vi "ttlpuls.vi"(0 "lines":tag="Dev1/port2/line7", 1 "Pause Time (ms)":u32=2000, 2 "Pulse Length (ms)":u32=300, 3 "Number of Pulses":i32=5) -> ()   [LabVIEW 2011]
uses:
  <vilib>/DAQmx/write.llb/DAQmx Write (Digital 1D Bool 1Chan 1Samp).vi
  <vilib>/DAQmx/create/channels.llb/DAQmx Create Channel (DO-Digital Output).vi
  <vilib>/DAQmx/miscellaneous.llb/DAQmx Fill In Error Info.vi
  Program Files/National Instruments/LabVIEW 2011/resource/objmgr/daqmx.rc
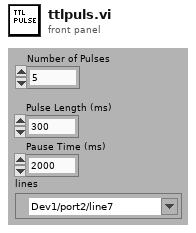
[diagram p1: front panel]
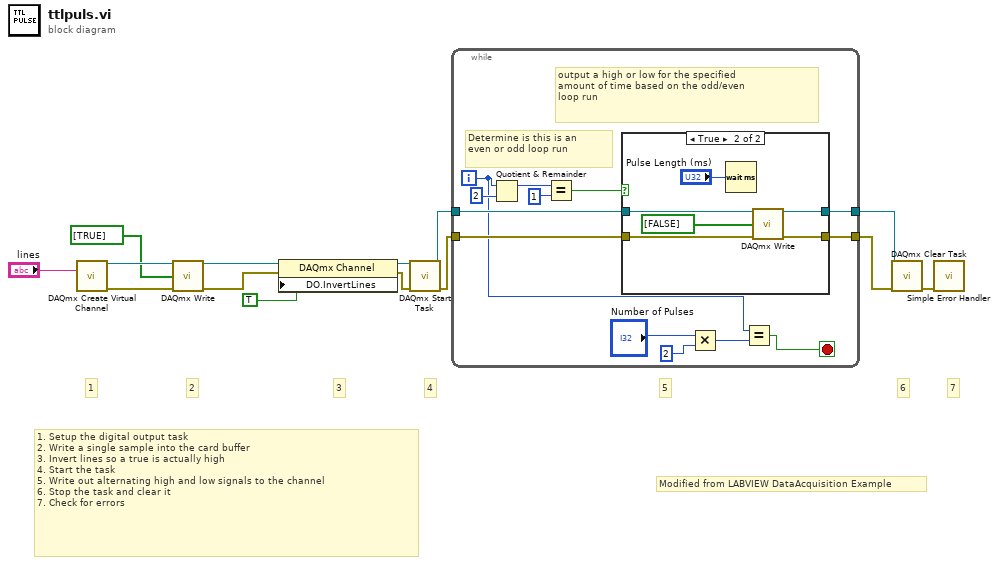
[diagram p0: block diagram]
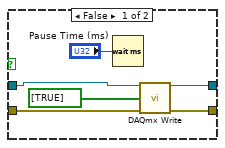
[diagram p2: hidden frame]
diagram:
  # "Modified from LABVIEW DataAcquisition Example"
  # "5"
  # "1. Setup the digital output task\n2. Write a single sample into the card buffer\n3. Invert lines so a true is actually high\n4. Start the task\n5. Write out alternating high and low signals to the channel\n6. Stop the task and clear it\n7. Check for errors"
  # "7"
  # "6"
  # "4"
  # "3"
  # "2"
  # "1"
  n1 = call-poly <vilib>:"DAQmx Create Virtual Channel.vi"("lines"="lines") -> ("task out"=w14:refnum<k21>, "error out"=w13:errorcluster)  [unwired: 13 in]
  n2 = call-poly <vilib>:"DAQmx Write.vi"("task/channels in"=w14, "data"=bool[] [TRUE], "error in"=w13) -> ("task out"=w5:refnum<k21>, "error out"=w1:errorcluster)  [unwired: 10 in, 1 out]
  n3 = property class="DAQmx Channel"(reference=w5, error in=w1, "DO.InvertLines"=TRUE) -> (reference out=w4:refnum<k21>, error out=w3:errorcluster)
  n4 = call <vilib>:"DAQmx Start Task.vi"("task/channels in"=w4, "error in"=w3) -> ("task out"=w12:refnum<k21>, "error out"=w11:errorcluster)  [unwired: 12 in]
  n5 = while {
    tunnel: w12 -> [w27]
    tunnel: w11 -> [w26]
    tunnel: [w25] -> w10
    tunnel: [w24] -> w9
    i -> [w18]
    stop <- w19 stop-if-true
    # "output a high or low for the specified\namount of time based on the odd/even\nloop run"
    # "Determine is this is an\neven or odd loop run"
    n6 = Quotient & Remainder(x=w18, y=2) -> (x-y*floor(x/y)=w22:i32)  [unwired: 1 out]
    n7 = Equal?(x=w22, y=1) -> (x = y?=w20:bool)
    n8 = case shown="True" w20 {
      tunnel: w27 -> [w31 w39]
      tunnel: w26 -> [w30 w38]
      tunnel: [w32 w37] -> w25
      tunnel: [w33 w36] -> w24
      frame False {
        n9 = Wait (ms)(milliseconds to wait="Pause Time (ms)") -> ()  [unwired: 1 out]
        n10 = call-poly <vilib>:"DAQmx Write.vi"("task/channels in"=w31, "data"=bool[] [TRUE], "error in"=w30) -> ("task out"=w33:refnum<k21>, "error out"=w32:errorcluster)  [unwired: 10 in, 1 out]
      }
      frame True {
        n11 = Wait (ms)(milliseconds to wait="Pulse Length (ms)") -> ()  [unwired: 1 out]
        n12 = call-poly <vilib>:"DAQmx Write.vi"("task/channels in"=w39, "data"=bool[] [FALSE], "error in"=w38) -> ("task out"=w36:refnum<k21>, "error out"=w37:errorcluster)  [unwired: 10 in, 1 out]
      }
    }
    n13 = Multiply(x="Number of Pulses", y=2) -> (x*y=w15:i32)
    n14 = Equal?(x=w18, y=w15) -> (x = y?=w19:bool)
  }
  n15 = call <vilib>:"DAQmx Clear Task.vi"("task in"=w9, "error in"=w10) -> ("error out"=w8:errorcluster)  [unwired: 13 in]
  n16 = call <vilib>:"Simple Error Handler.vi"("error in (no error)"=w8) -> ()  [unwired: 4 in, 5 out]
